vi "Request_str_JSON.vi"(0 "reference in":T1, 5 "method":string, 7 "params":refnum<class "JSON Null.lvclass">, 9 "id":string, 11 "error in (no error)":errorcluster) -> (4 "reference out":T1, 6 "JSON out":refnum<class "JSON Null.lvclass">, 15 "error out":errorcluster)   [LabVIEW 2017, in "JSON_RPC_client.lvlib"]
uses:
  JSON_RPC_client.lvlib
  reference.ctl
  <vilib>/httpClient/ClientHandle.ctl
  <vilib>/NI/JSON Support for LabVIEW/JSON Data Classes/JSON Datatype/JSON Null.lvclass
  <vilib>/NI/JSON Support for LabVIEW/JSON Data Classes/JSON Object/New JSON Object (Empty).vi
  <vilib>/NI/JSON Support for LabVIEW/JSON Data Classes/JSON Object/Insert Key Value Pair.vi
  <vilib>/NI/JSON Support for LabVIEW/JSON Data Classes/JSON Object/Insert Key Value Pair (Single String).vi
  <vilib>/NI/JSON Support for LabVIEW/JSON Data Classes/JSON Object/Insert Key Value Pair (Single).vi
  <vilib>/httpClient/POSTBuffer.vi
  <vilib>/NI/JSON Support for LabVIEW/JSON Data Classes/JSON Helper/Parsing/Parse Value.vi
  <vilib>/NI/JSON Support for LabVIEW/JSON Data Classes/JSON Object/Set Object Parameters XNode/Set Object Parameters.xnode
  <vilib>/NI/JSON Support for LabVIEW/JSON Data Classes/JSON Object/JSON Object.lvclass
  <vilib>/httpClient/LabVIEWHTTPClient.lvlib
  <vilib>/NI/JSON Support for LabVIEW/JSON Data Classes/JSON Helper/JSON Helper.lvclass
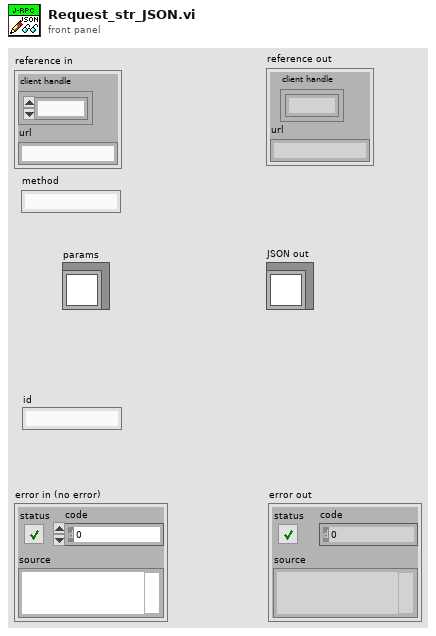
[diagram p1: front panel]
types:
  T1 = typedef "JSON_RPC_client.lvlib/reference.ctl" = cluster{"client handle":T2, "url":string}
  T2 = typedef "LabVIEWHTTPClient.lvlib/ClientHandle.ctl" = refnum<k1>
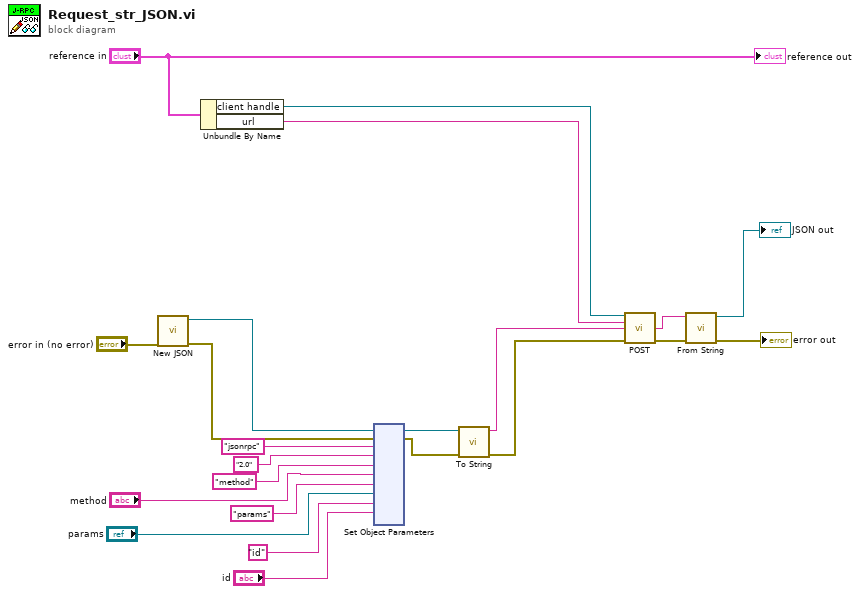
[diagram p0: block diagram]
diagram:
  n1 = call-poly <vilib>:"New JSON.vi"("error in (no error)"="error in (no error)") -> ("error out"=w12:errorcluster, "JSON Object out"=w13:refnum<class "JSON Object.lvclass">)  [unwired: 9 in]
  n2 = Unbundle By Name("reference in") -> ("client handle"=w21:T2, "url"=w20:string)
  n3 = xnode "Set Object Parameters"("key"="jsonrpc" ("Name"), "key"="method" ("Name"), "key"="params" ("Name"), "key"="id" ("Name"), "parameter"="2.0" ("String"), "parameter"="method", "parameter"="params", "parameter"="id", "JSON Object In"=w13, "error in"=w12) -> ("JSON Object Out"=w4:refnum<class "JSON Object.lvclass">, "error out"=w3:errorcluster)  [unwired: 4 out]
  n4 = call-dynamic "To String.vi"("error in (no error)"=w3, "JSON Object in"=w4) -> ("error out"=w1:errorcluster, "String"=w2:string)  [unwired: 8 in]
  n5 = call-poly <vilib>:"POST.vi"("client handle"=w21, "url"=w20, "buffer"=w2, "error in (no error)"=w1) -> ("body"=w17:string, "error out"=w18:errorcluster)  [unwired: 8 in, 2 out]
  n6 = call <vilib>:"From String.vi"("error in (no error)"=w18, "JSON String"=w17) -> ("error out"=→"error out":errorcluster, "JSON out"=→"JSON out":refnum<class "JSON Null.lvclass">)  [unwired: 8 in]
  "reference out" <- "reference in"
